vi "PECT_Feature extraction.vi"(6 "Length T/2":i32=50, 7 "Offset":bool, 8 "Length":i32=50, 9 "Start 2":i32=50, 10 "Start 1":i32, 11 "Pulse signal in":dbl[](array[numeric])) -> (3 "Feature extraction out":dbl)   [LabVIEW 2018]
uses:
  <vilib>/measure/maspectr.llb/FFT Power Spectrum and PSD for 1 Chan.vi
  <vilib>/measure/NI_MAPro.lvlib
panel:
  out "PSD":dbl[](graph)
  in  "delta t (s)":dbl=1.25e-06
  in  "End idx":i32=2000
  in  "Start idx":i32
  out "Filter":dbl[](graph)
  out "dX":dbl[](graph)
  out "Original":dbl[](graph)
  out "Feature extraction graph":dbl(graph)
  # "Start 1: data index at Gate 1\nStart 2: data index at Gate 2\nLength = Start 2 - Start 1\nLength T/2 = half length of 1 pulse\nOffset: remove offset data"
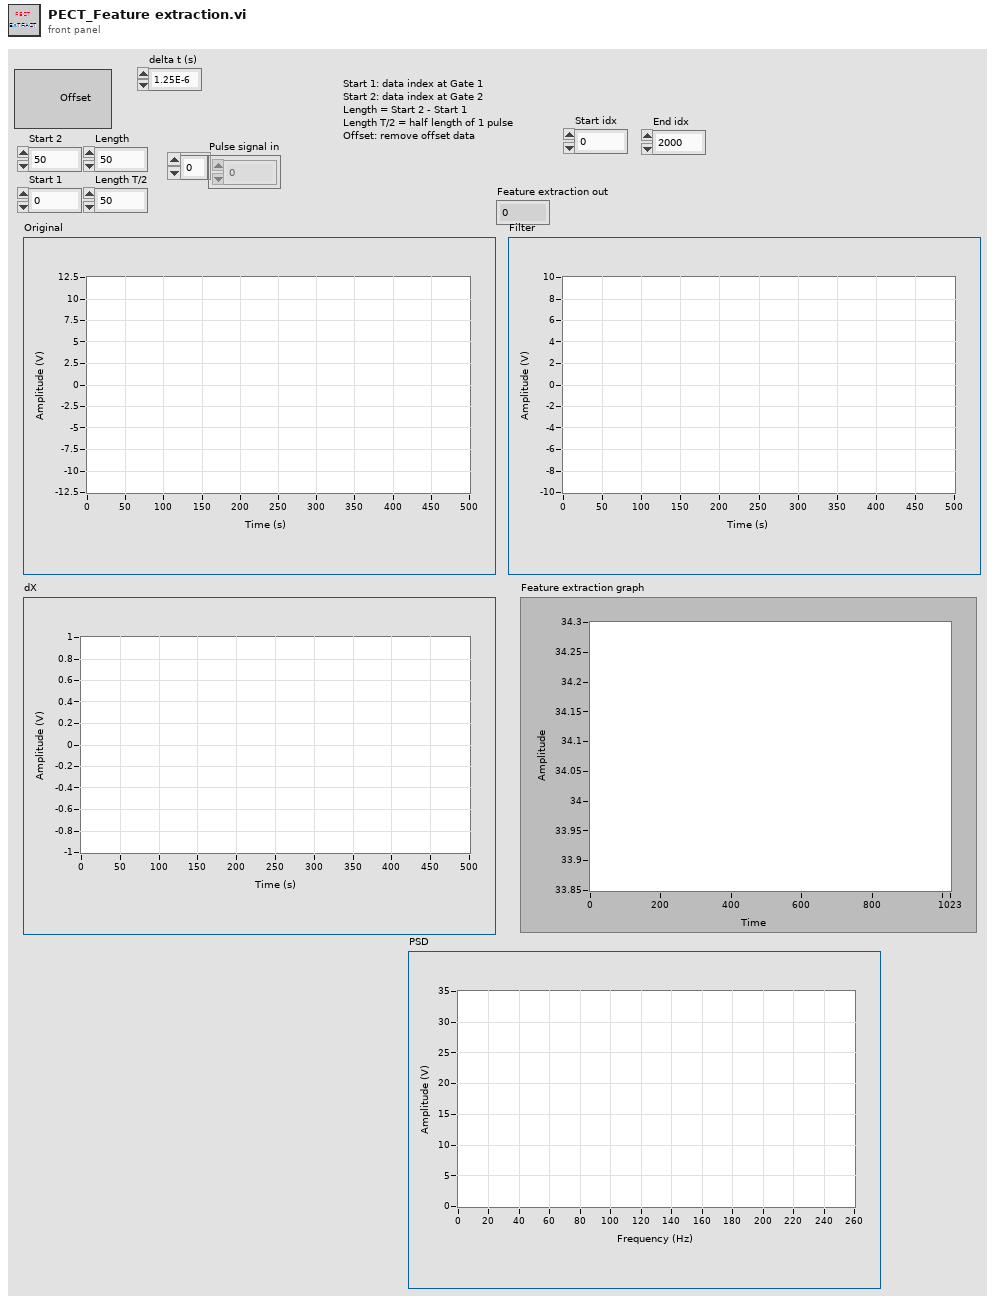
[diagram p1: front panel]
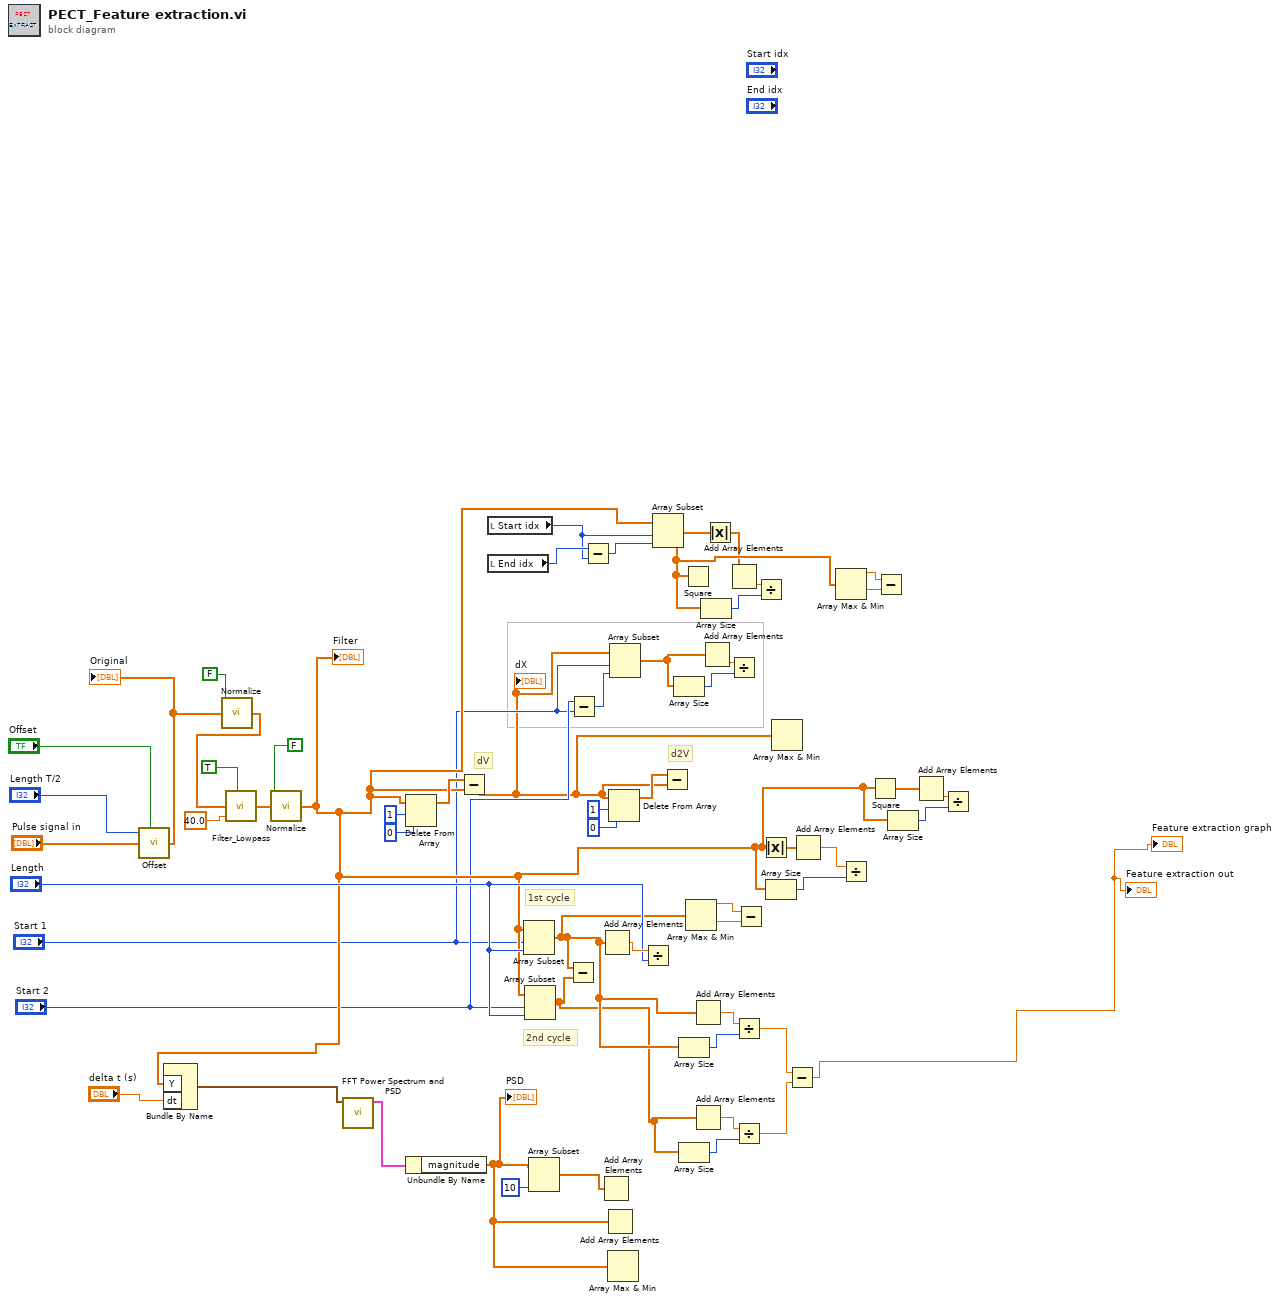
[diagram p0: block diagram]
diagram:
  # "d2V"
  # "dV"
  # "2nd cycle"
  # "1st cycle"
  n1 = call "Offset.vi"("Length T/2"="Length T/2", "Offset"="Offset", "Pulse signal in"="Pulse signal in") -> ("Pulse signal out"=w19:dbl[])  [unwired: 4 in]
  "Original" <- w19
  n2 = call "Normalize.vi"("Normalization"=FALSE, "Pulse signal in"=w19) -> ("Pulse signal out"=w18:dbl[])  [unwired: 5 in]
  n3 = call "Filter_Lowpass.vi"("Filter"=TRUE, "Pulse signal in"=w18, "low cutoff freq: fl"=40.0) -> ("Signal out"=w24:dbl[])  [unwired: 6 in]
  n4 = call "Normalize.vi"("Normalization"=FALSE, "Pulse signal in"=w24) -> ("Pulse signal out"=w12:dbl[])  [unwired: 5 in]
  "Filter" <- w12
  n5 = Bundle By Name("Y"=w12, "dt"="delta t (s)") -> (w29:waveform(dbl))  [unwired: 1 in]
  n6 = call-poly <vilib>:"FFT Power Spectrum and PSD.vi"("time signal"=w29) -> ("Power Spectrum / PSD"=w28:cluster{"f0":dbl, "df":dbl, "magnitude":dbl[]})  [unwired: 7 in, 3 out]
  n7 = Delete From Array(array=w12, length=1, index=0) -> (array with subset deleted=w56:dbl[])  [unwired: 1 out]
  n8 = Unbundle By Name(w28) -> ("magnitude"=w27:dbl[])
  "PSD" <- w27
  n9 = Subtract(x=w56, y=w12) -> (x-y=w5:dbl[])
  "dX" <- w5
  n10 = local read "Start idx"() -> (w39:i32)
  n11 = local read "End idx"() -> (w43:i32)
  n12 = Array Subset(array=w12, index="Start 1", length="Length") -> (w10:dbl[])
  n13 = Array Subset(array=w12, index="Start 2", length="Length") -> (w9:dbl[])
  n14 = Array Subset(array=w27, length=10) -> (w25:dbl[])  [unwired: 1 in]
  n15 = Subtract(x=w10, y=w9) -> ()  [unwired: 1 out]
  n16 = Subtract(x="Start 2", y="Start 1") -> (x-y=w7:i32)
  n17 = Subtract(x=w43, y=w39) -> (x-y=w40:i32)
  n18 = Add Array Elements(numeric array=w25) -> ()  [unwired: 1 out]
  n19 = Add Array Elements(numeric array=w10) -> (sum=w53:dbl)
  n20 = Add Array Elements(numeric array=w27) -> ()  [unwired: 1 out]
  n21 = Array Max & Min(array=w27) -> ()  [unwired: 4 out]
  n22 = Delete From Array(array=w5, length=1, index=0) -> (array with subset deleted=w48:dbl[])  [unwired: 1 out]
  n23 = Array Subset(array=w5, index="Start 1", length=w7) -> (w2:dbl[])
  n24 = Divide(x=w53, y="Length") -> ()  [unwired: 1 out]
  n25 = Array Subset(array=w12, index=w39, length=w40) -> (w17:dbl[])
  n26 = Subtract(x=w48, y=w5) -> ()  [unwired: 1 out]
  n27 = Array Size(array=w2) -> (size(s)=w3:i32)
  n28 = Array Size(array=w10) -> (size(s)=w35:i32)
  n29 = Array Size(array=w9) -> (size(s)=w32:i32)
  n30 = Square(x=w17) -> ()  [unwired: 1 out]
  n31 = Array Max & Min(array=w10) -> (max value=w23:dbl, min value=w49:dbl)  [unwired: 2 out]
  n32 = Add Array Elements(numeric array=w10) -> (sum=w34:dbl)
  n33 = Add Array Elements(numeric array=w9) -> (sum=w33:dbl)
  n34 = Array Size(array=w17) -> (size(s)=w41:i32)
  n35 = Add Array Elements(numeric array=w2) -> (sum=w4:dbl)
  n36 = Absolute Value(x=w17) -> (abs(x)=w16:dbl[])
  n37 = Add Array Elements(numeric array=w16) -> (sum=w42:dbl)
  n38 = Divide(x=w4, y=w3) -> ()  [unwired: 1 out]
  n39 = Divide(x=w34, y=w35) -> (x/y=w11:dbl)
  n40 = Divide(x=w33, y=w32) -> (x/y=w31:dbl)
  n41 = Subtract(x=w23, y=w49) -> ()  [unwired: 1 out]
  n42 = Divide(x=w42, y=w41) -> ()  [unwired: 1 out]
  n43 = Absolute Value(x=w12) -> (abs(x)=w36:dbl[])
  n44 = Array Size(array=w12) -> (size(s)=w38:i32)
  n45 = Array Max & Min(array=w5) -> ()  [unwired: 4 out]
  n46 = Subtract(x=w11, y=w31) -> (x-y=→"Feature extraction graph" →"Feature extraction out":dbl)
  n47 = Add Array Elements(numeric array=w36) -> (sum=w37:dbl)
  n48 = Array Max & Min(array=w17) -> (max value=w22:dbl, min value=w21:dbl)  [unwired: 2 out]
  n49 = Divide(x=w37, y=w38) -> ()  [unwired: 1 out]
  n50 = Square(x=w12) -> (x^2=w13:dbl[])
  n51 = Subtract(x=w22, y=w21) -> ()  [unwired: 1 out]
  n52 = Array Size(array=w12) -> (size(s)=w15:i32)
  n53 = Add Array Elements(numeric array=w13) -> (sum=w14:dbl)
  n54 = Divide(x=w14, y=w15) -> ()  [unwired: 1 out]
